vi "GetMSGName.vi"(11 "MC-ExternClientInterface in":refnum<class "MC-ExternClientInterface.lvclass">) -> (2 "NAME":string, 3 "MC-ExternClientInterface out":refnum<class "MC-ExternClientInterface.lvclass">)   [LabVIEW 2020, in "MC-ExternClient.lvlib" / "MC-ExternClientInterface.lvclass"]
uses:
  MC-ExternClientInterface.lvclass
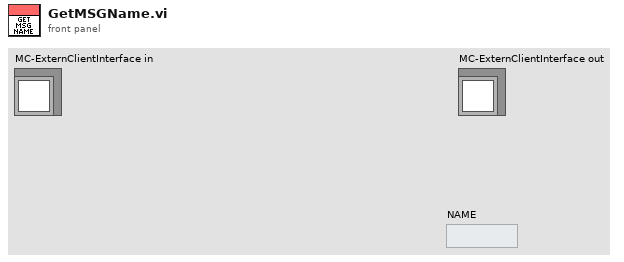
[diagram p1: front panel]
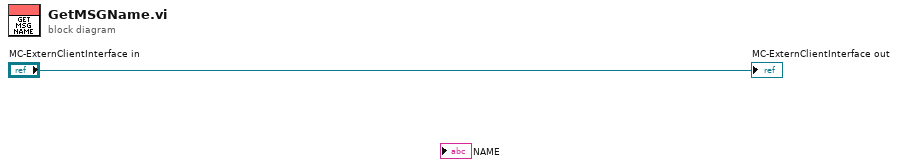
[diagram p0: block diagram]
diagram:
  "MC-ExternClientInterface out" <- "MC-ExternClientInterface in"
